vi "Full_Power_Setting.vi"(8 "error in (no error)":errorcluster, 10 "Vesta in":refnum<queue>, 11 "Data Cluster In":T1 {"VestaTemperature"."Water Heater Temp (°F)" min=32 max=203}) -> (0 "error out":errorcluster, 3 "Data Cluster Out":T1 {"VestaTemperature"."Water Heater Temp (°F)" min=32 max=203})   [LabVIEW 2023]
uses:
  Message Queue/Message Queue.lvlib
  Message Queue/Enqueue Message (Single).vi
  Drivers/Resideo Gas Valve/Type Definitions/Temperature Control.ctl
  Message Queue/Message Cluster.ctl
  Drivers/Resideo Gas Valve/Type Definitions/Vesta Info.ctl
  controls/Burner Duty Cycle.ctl
  controls/Timer Application Cluster.ctl
  controls/UI Data.ctl
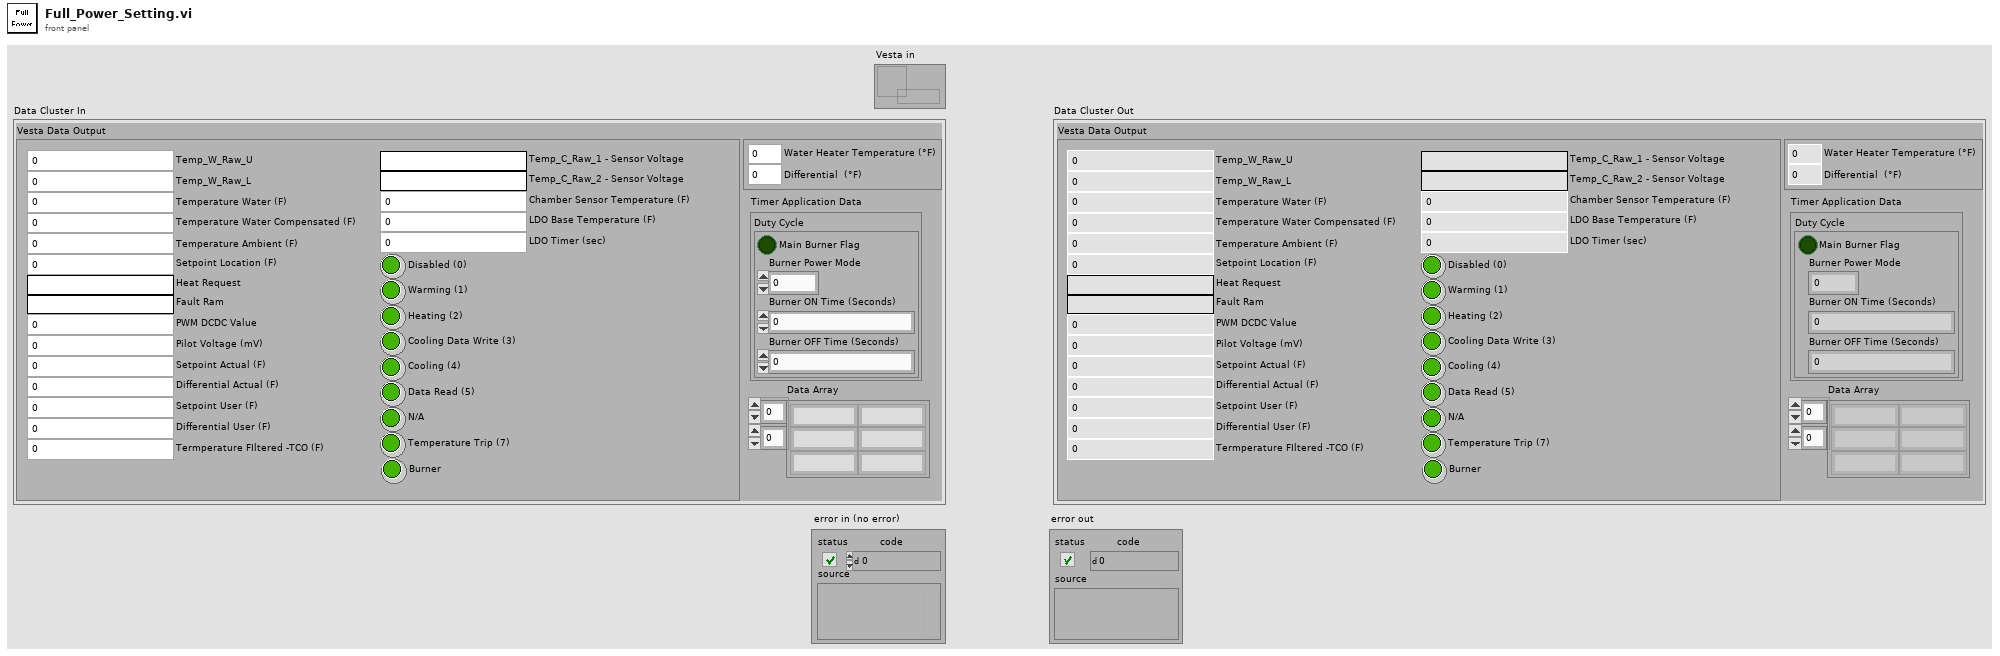
[diagram p1: front panel]
types:
  T1 = typedef "UI Data.ctl" = cluster{"Vesta Data Output":T2, "VestaTemperature":T3, "Timer Application Data":T4, "Data Array":string[][]}
  T2 = typedef "Vesta Info.ctl" = cluster{"Temp_W_Raw_U":u16, "Temp_W_Raw_L":u16, "Temperature Water (F)":dbl, "Temperature Water Compensated (F)":dbl, "Temperature Ambient (F)":dbl, "Setpoint Location (F)":dbl, "Heat Request":string, "Fault Ram":string, "PWM DCDC Value":u16, "Pilot Voltage (mV)":dbl, "Setpoint Actual (F)":dbl, "Differential Actual (F)":dbl, "Setpoint User (F)":dbl, "Differential User (F)":dbl, "Termperature FIltered -TCO (F)":dbl, "Temp_C_Raw_1 - Sensor Voltage":string, "Temp_C_Raw_2 - Sensor Voltage":string, "Chamber Sensor Temperature (F)":dbl, "LDO Base Temperature (F)":dbl, "LDO Timer (sec)":i16, "Disabled (0)":bool, "Warming (1)":bool, "Heating (2)":bool, "Cooling Data Write (3)":bool, "Cooling (4)":bool, "Data Read (5)":bool, "N/A":bool, "Temperature Trip (7)":bool, "Burner":bool}
  T3 = typedef "Temperature Control.ctl" = cluster{"Water Heater Temp (°F)":u16, "Differential  (°F)":dbl}
  T4 = typedef "Timer Application Cluster.ctl" = cluster{"Duty Cycle":T5}
  T5 = typedef "Burner Duty Cycle.ctl" = cluster{"Burner ON Time (Seconds)":dbl, "Burner OFF Time (Seconds)":dbl, "Main Burner Flag":bool, "Burner Power Mode":u8}
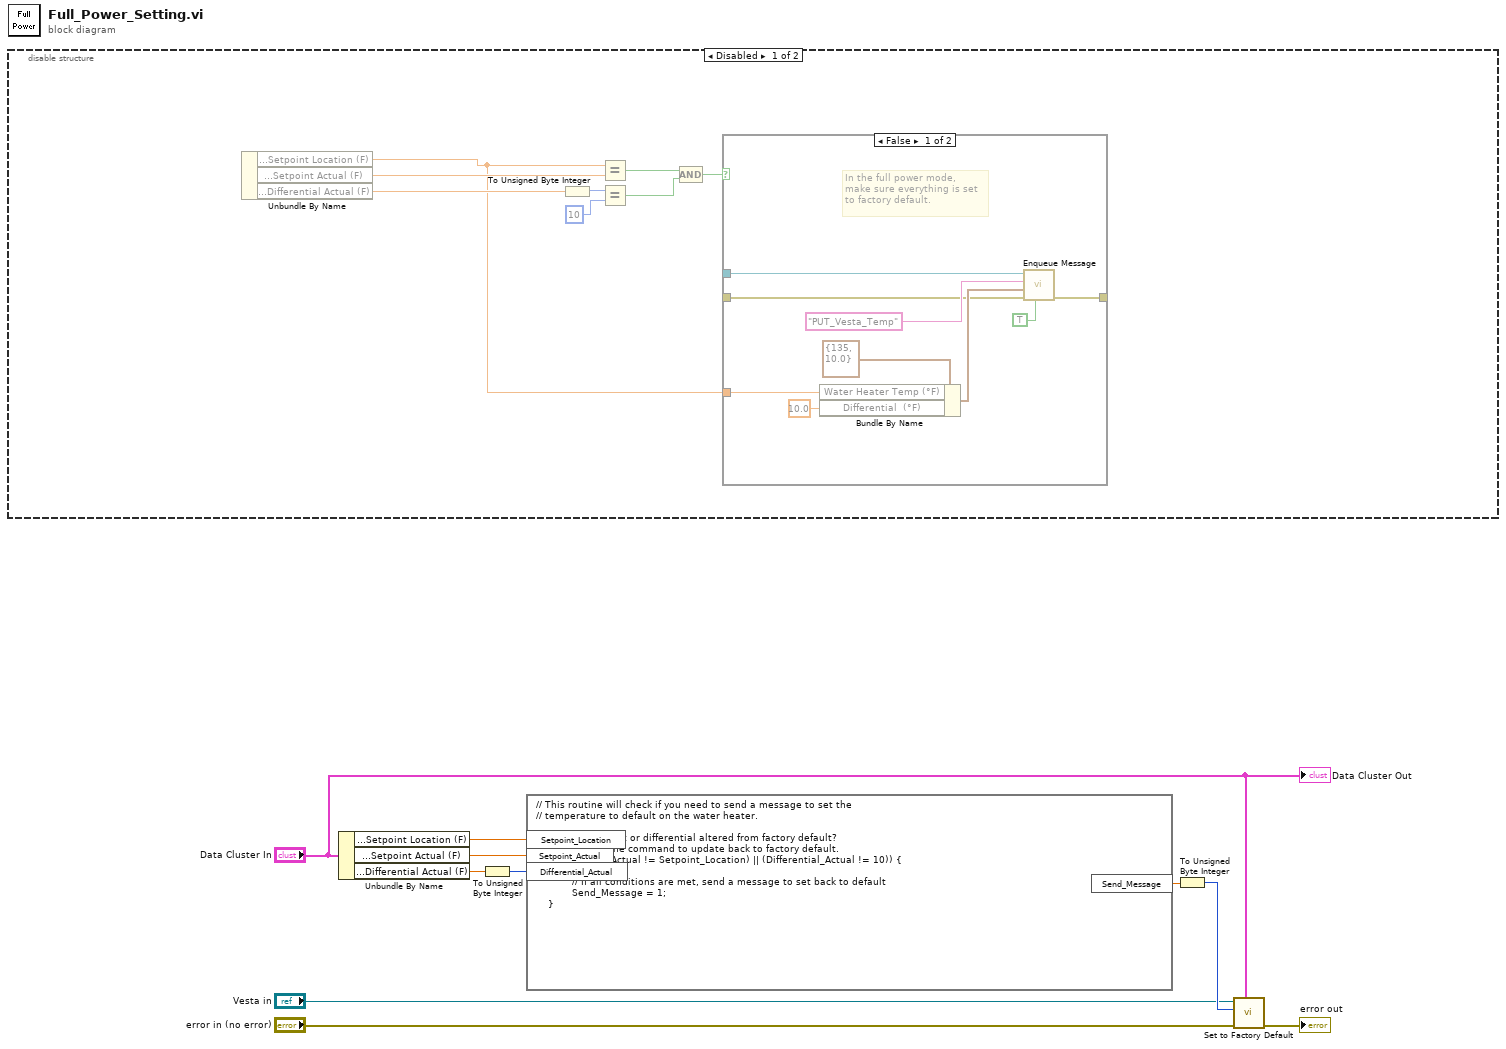
[diagram p0: block diagram]
diagram:
  n1 = disable-structure shown="Disabled" {
    frame Disabled {
      n2 = Unbundle By Name() -> ("Vesta Data Output.Setpoint Location (F)"=w11:dbl, "Vesta Data Output.Setpoint Actual (F)"=w15:dbl, "Vesta Data Output.Differential Actual (F)"=w16:dbl)  [unwired: 1 in]
      n3 = To Unsigned Byte Integer(number=w16) -> (unsigned 8bit integer=w18:u8)
      n4 = Equal?(x=w11, y=w15) -> (x = y?=w13:bool)
      n5 = Equal?(x=w18, y=u8 10) -> (x = y?=w14:bool)
      n6 = Compound Arithmetic op=AND(w13, w14) -> (w12:bool)
      n7 = case shown="False" w12 {
        tunnel: _ -> [w22 _]
        tunnel: _ -> [w21 w28]
        tunnel: [w20 w28] -> _
        tunnel: w11 -> [w19 _]
        frame False {
          # "In the full power mode,\nmake sure everything is set\nto factory default."
          n8 = Bundle By Name(cluster=T3 {"Water Heater Temp (°F)"=135, "Differential  (°F)"=10.0} ("VestaTemperature"), "Water Heater Temp (°F)"=w19, "Differential  (°F)"=10.0) -> (w27:T3)
          n9 = call-poly "Enqueue Message.vi"("Priority Message? (F)"=TRUE, "error in (no error)"=w21, "Message Data"=w27, "Message"="PUT_Vesta_Temp", "Message Queue"=w22) -> ("error out"=w20:errorcluster)  [unwired: 5 in, 1 out]
        }
        frame True {
          # "If the settings are correct, no\nneed to send them again."
        }
      }
    }
    frame Enabled {
    }
  }
  n10 = Unbundle By Name("Data Cluster In") -> ("Vesta Data Output.Setpoint Location (F)"=w10:dbl, "Vesta Data Output.Setpoint Actual (F)"=w9:dbl, "Vesta Data Output.Differential Actual (F)"=w8:dbl)
  n11 = To Unsigned Byte Integer(number=w8) -> (unsigned 8bit integer=w7:u8)
  n12 = formula code="// This routine will check if you need to send a message to set the \n// temperature to default on the water heater.\n    \n    // Is the setpoint or differential altered from factory default?\n    // If so, send the command to update back to factory default.\n    if ((Setpoint_Actual != Setpoint_Location) || (Differential_Actual != 10)) {             \n            \n            // If all conditions are met, send a message to set back to default\n            Send_Message = 1;  \n    }"("Setpoint_Actual"=w9, "Setpoint_Location"=w10, "Differential_Actual"=w7) -> ("Send_Message"=w6:dbl)
  n13 = To Unsigned Byte Integer(number=w6) -> (unsigned 8bit integer=w5:u8)
  n14 = call "Set to Factory Default.vi"(7:"Data Cluster In", "error in (no error)"="error in (no error)", "Vesta in"=w5, "Data Cluster In"="Vesta in") -> ("error out"=→"error out":errorcluster)  [unwired: 6 in, 1 out]
  "Data Cluster Out" <- "Data Cluster In"
